vi "Operational.vi"(8 "error in (no error)":errorcluster, 11 "Instrument in":refnum<class "Instrument.lvclass">) -> (0 "error out":errorcluster, 3 "Instrument out":refnum<class "Instrument.lvclass">)   [LabVIEW 2018, in "Instrument.lvclass"]
uses:
  Instrument.lvclass
  C:/Users/devstaff/sparc4/s4gui/Versao ZeroMQ REQ-REP/SPARC4_GUI -v1.0.0 - 20250122_ICS-JSON/Server/Server.lvclass
  Server/Server.lvclass/Server.ctl
  Instrument.lvclass/Instrument.ctl
  Device/Optics/Optics.lvclass/Optics.ctl
  Device/Optics/Opt_Selector/Opt_Selector.lvclass
  C:/Users/devstaff/sparc4/s4gui/Versao ZeroMQ REQ-REP/SPARC4_GUI -v1.0.0 - 20250122_ICS-JSON/Device/Optics/Optics.lvclass
  Device/Optics/Opt_Continuous/Opt_Continuous.lvclass
  Server/Server.lvclass
  Device/Optics/Optics.lvclass
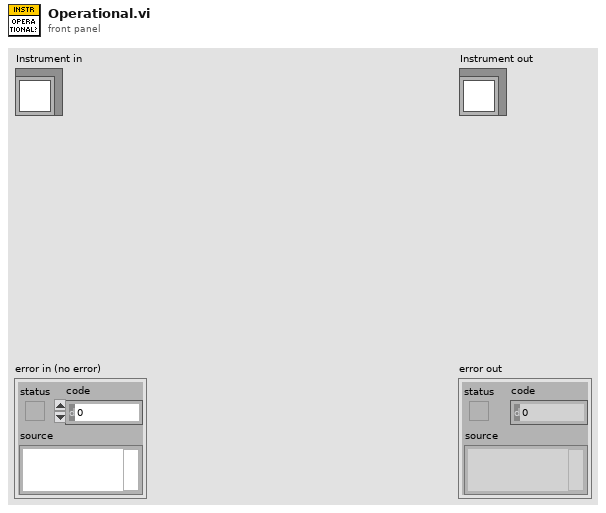
[diagram p1: front panel]
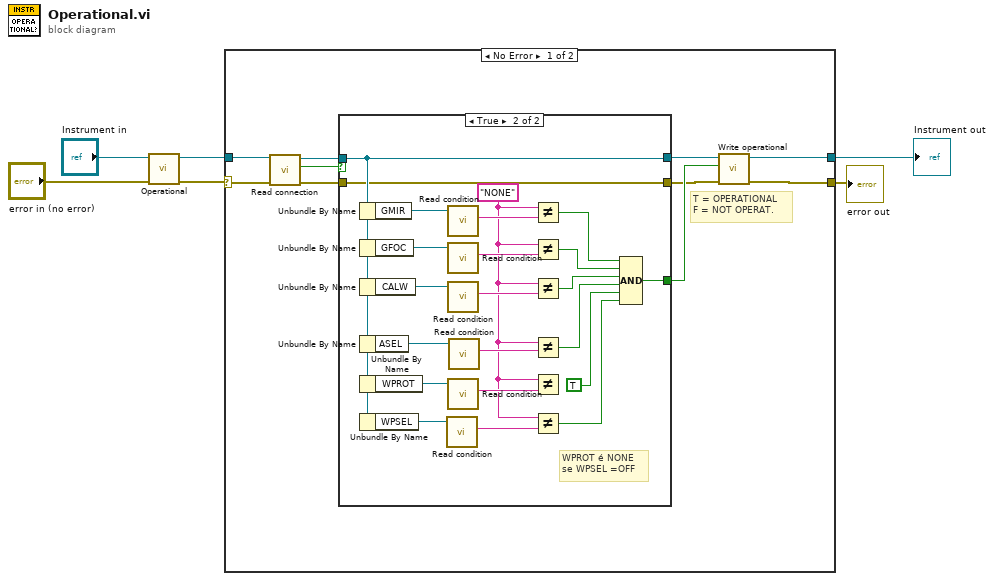
[diagram p0: block diagram]
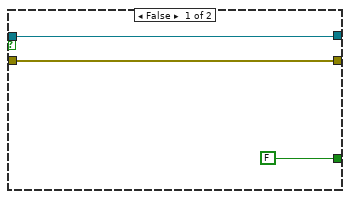
[diagram p2: hidden frame]
diagram:
  n1 = call-parent "Operational.vi"("error in (no error)"="error in (no error)", "Server in"="Instrument in") -> ("error out"=w4:errorcluster, "Server out"=w3:refnum<class "Instrument.lvclass">)  [unwired: 8 in]
  n2 = case shown="No Error" w4 {
    selector: w4 -> [w12 w42]
    tunnel: w3 -> [w13 w43]
    tunnel: [w14 w43] -> w1
    tunnel: [w15 w42] -> w2
    frame No Error {
      # "T = OPERATIONAL\nF = NOT OPERAT."
      n3 = call "Read connection.vi"("error in (no error)"=w12, "Server in"=w13) -> ("error out"=w9:errorcluster, "connection"=w7:bool, "Server out"=w11:refnum<class "Instrument.lvclass">)  [unwired: 7 in]
      n4 = case shown="True" w7 {
        tunnel: [FALSE w23] -> w16
        tunnel: w11 -> [w19 w22]
        tunnel: [w19 w22] -> w10
        tunnel: [w18 w21] -> w8
        tunnel: w9 -> [w18 w21]
        frame False {
        }
        frame True {
          w29 = "NONE"
          # "WPROT é NONE\nse WPSEL =OFF"
          n5 = Unbundle By Name(w22) -> ("GMIR"=w41:refnum<class "Opt_Continuous.lvclass">)
          n6 = Unbundle By Name(w22) -> ("GFOC"=w40:refnum<class "Opt_Continuous.lvclass">)
          n7 = Unbundle By Name(w22) -> ("CALW"=w39:refnum<class "Opt_Selector.lvclass">)
          n8 = Unbundle By Name(w22) -> ("ASEL"=w38:refnum<class "Opt_Selector.lvclass">)
          n9 = Unbundle By Name(w22) -> ("WPROT"=w37:refnum<class "Opt_Selector.lvclass">)
          n10 = Unbundle By Name(w22) -> ("WPSEL"=w36:refnum<class "Opt_Selector.lvclass">)
          n11 = call "Read condition.vi"("Optics in"=w36) -> ("condition"=w30:string)  [unwired: 8 in, 2 out]
          n12 = call "Read condition.vi"("Optics in"=w41) -> ("condition"=w35:string)  [unwired: 8 in, 2 out]
          n13 = call "Read condition.vi"("Optics in"=w40) -> ("condition"=w34:string)  [unwired: 8 in, 2 out]
          n14 = call "Read condition.vi"("Optics in"=w39) -> ("condition"=w33:string)  [unwired: 8 in, 2 out]
          n15 = call "Read condition.vi"("Optics in"=w37) -> ("condition"=w31:string)  [unwired: 8 in, 2 out]
          n16 = call "Read condition.vi"("Optics in"=w38) -> ("condition"=w32:string)  [unwired: 8 in, 2 out]
          n17 = Not Equal?(x=w29, y=w35) -> (x != y?=w28:bool)
          n18 = Not Equal?(x=w29, y=w34) -> (x != y?=w27:bool)
          n19 = Not Equal?(x=w29, y=w33) -> (x != y?=w26:bool)
          n20 = Not Equal?(x=w29, y=w32) -> (x != y?=w25:bool)
          n21 = Not Equal?(x=w29, y=w31) -> ()  [unwired: 1 out]
          n22 = Not Equal?(x=w29, y=w30) -> (x != y?=w24:bool)
          n23 = Compound Arithmetic op=AND(w28, w27, w26, w25, TRUE ("value"), w24) -> (w23:bool)
        }
      }
      n24 = call-dynamic "Write operational.vi"("error in (no error)"=w8, "operational"=w16, "Server in"=w10) -> ("error out"=w15:errorcluster, "Server out"=w14:refnum<class "Instrument.lvclass">)  [unwired: 7 in]
    }
    frame Error {
    }
  }
  "error out" <- w2
  "Instrument out" <- w1
